vi "OPTIONS.vi"(6 "timeout":i32=10000, 7 "output file":path, 8 "error in":errorcluster, 10 "url":string, 11 "Session In":refnum<class "Session.lvclass">) -> (0 "error out":errorcluster, 1 "body":string, 2 "headers":string, 3 "Session Out":refnum<class "Session.lvclass">, 4 "status code":u32)   [LabVIEW 2020, in "Library Commun.lvlib" / "Library Http.lvlib" / "Session.lvclass"]
doc: "Sends a web request returning headers and body data from a server, web page, or web service. This VI uses the OPTIONS HTTP method and does not submit any data to the server."
uses:
  Session.lvclass
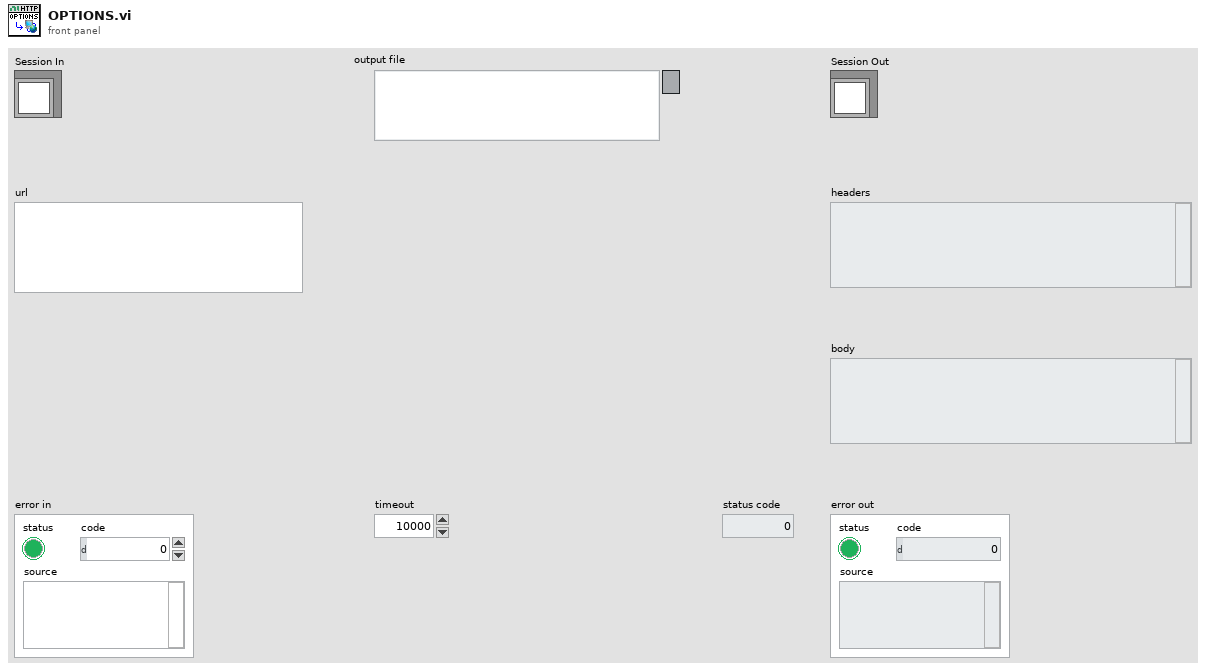
[diagram p1: front panel]
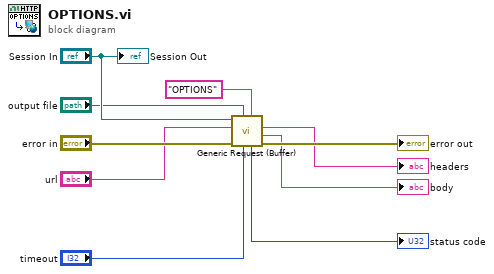
[diagram p0: block diagram]
diagram:
  n1 = call "Generic Request (Buffer).vi"("method"="OPTIONS", "timeout"="timeout", "output file"="output file", "error in"="error in", "url"="url", "Session In"="Session In") -> ("error out"=→"error out":errorcluster, "body"=→"body":string, "headers"=→"headers":string, "status code"=→"status code":u32)  [unwired: 1 in, 1 out]
  "Session Out" <- "Session In"
